vi "Test Assert Update Event to JSON.vi"(10 "Assert Update":T1) -> (2 "<JSON>Assertion Update Event":string)   [LabVIEW 2013, in "Caraya.lvlib" / "Test Result.lvclass"]
uses:
  Test Result.lvclass
  Test Verbose Explanation.ctl
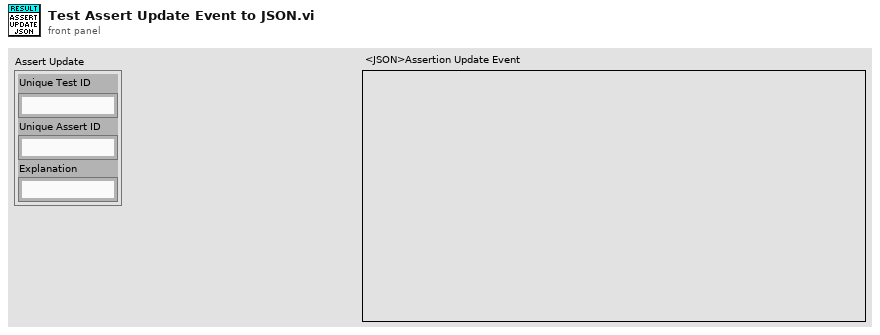
[diagram p1: front panel]
types:
  T1 = typedef "Caraya.lvlib/Test Result.lvclass/Test Verbose Explanation.ctl" = cluster{"Unique Test ID":string, "Unique Assert ID":string, "Explanation":string}
  T2 = cluster{"assert-id":string, "explanation":string}
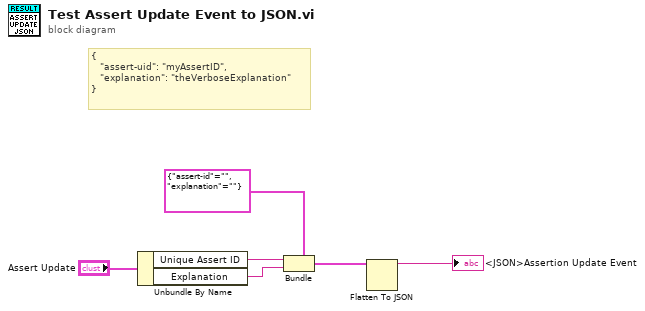
[diagram p0: block diagram]
diagram:
  # "{\n   \"assert-uid\": \"myAssertID\",\n   \"explanation\": \"theVerboseExplanation\"\n}"
  n1 = Unbundle By Name("Assert Update") -> ("Unique Assert ID"=w4:string, "Explanation"=w1:string)
  n2 = Bundle(cluster=T2 {"assert-id"="", "explanation"=""}, "assert-id"=w4, "explanation"=w1) -> (w5:T2)
  n3 = Flatten To JSON(anything=w5) -> (JSON string=→"<JSON>Assertion Update Event":string)  [unwired: 2 in, 1 out]
